vi "Test Micron Driver.vi"() -> ()   [LabVIEW 2024]
uses:
  Micron optics didgitizer configuration.ctl
  Micron Optics Driver/Micron Optics Driver.lvclass
  C:/Git/NHMFL_Core/Libraries/Instruments/VISA Instrument/VISA Instrument.lvclass
  C:/Git/NHMFL_Core/Libraries/Instruments/Instrument Driver/Instrument Driver.lvclass
  Micron sm Digitizer/Micron sm Digitizer.lvclass
  C:/Git/NHMFL_Core/Libraries/Instruments/Micron Optics/Micron Optics Driver/Micron Optics Driver.lvclass
  Micron Hyperion Driver/Micron Hyperion Driver.lvclass
  VISA Instrument/VISA Instrument.lvclass/VISA Instrument.ctl
  Instrument Driver/Instrument Driver.lvclass/Instrument Driver.ctl
  VISA Instrument/Write VISA resource.vi
  Instrument Driver/Write Cycle period.vi
panel:
  out "Waveform Chart":dbl[][](graph)
  in  "Micron Optics Digitizer Configuration":T1={"Post-trigger delay"=0.01, "Post-trigger duration"=0.1, "Rate"=1000000.0, "Reference channel"=-1, "Detection Setting IDs"=[130, 130], "Stream and average"=FALSE, "Address"="10.0.0.55"} {"Rate" format="%#_8pHz"; "Post-trigger duration" format="%#_6ps"; "Post-trigger delay" format="%#_6ps"}
  in  "sm-130  VISA resource":refnum<visa-resource-name>
  in  "Model":enum16{"NONE", "sm-130", "Hyperion"}(ring)=enum."sm-130"
  out "Channel names":string[](array[string])
  in  "stop":bool
  in  "milliseconds to wait":u32=1000
  in  "error in (no error)":errorcluster
  # "Pulse config"
  # "Monitor config"
  # "CH1\n.\n.\n.\n.\n.\nCH4"
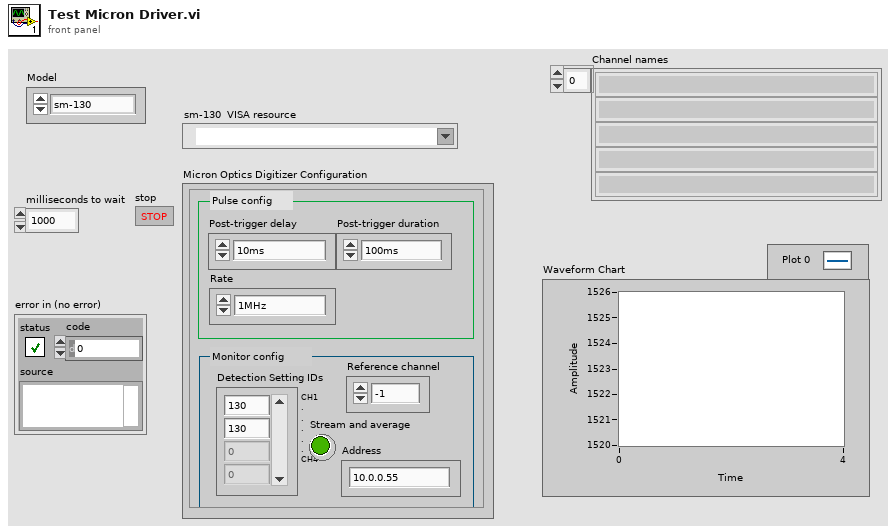
[diagram p1: front panel]
types:
  T1 = typedef "Micron optics didgitizer configuration.ctl" = cluster{"Post-trigger delay":dbl, "Post-trigger duration":dbl, "Rate":dbl, "Reference channel":i32, "Detection Setting IDs":u8[], "Stream and average":bool, "Address":string}
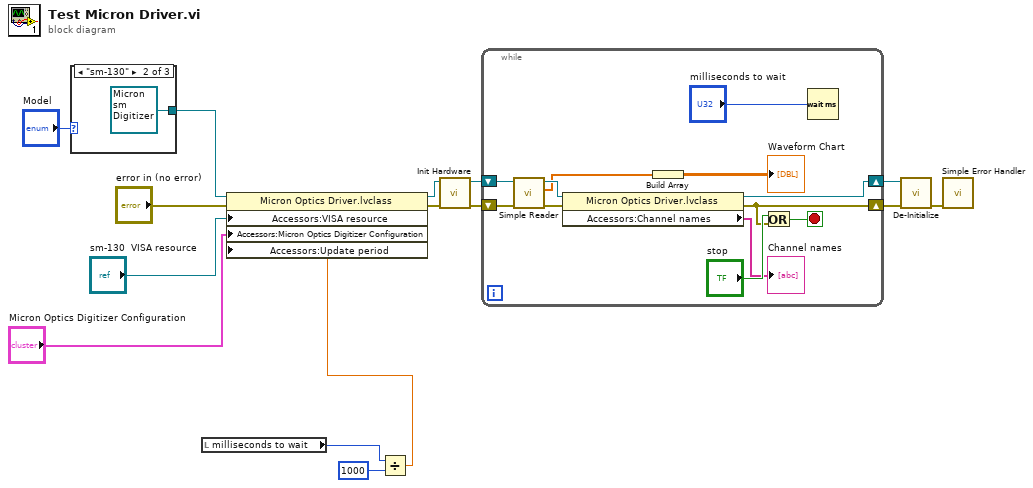
[diagram p0: block diagram]
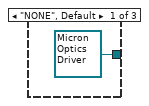
[diagram p2: hidden frame]
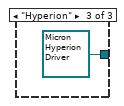
[diagram p3: hidden frame]
diagram:
  n1 = case shown="\"sm-130\"" "Model" {
    tunnel: [refnum<class "Micron Optics Driver.lvclass"> refnum ("Micron Optics Driver.lvclass") refnum<class "Micron sm Digitizer.lvclass"> refnum ("Micron sm Digitizer.lvclass") refnum<class "Micron Hyperion Driver.lvclass"> refnum ("Micron Hyperion Driver.lvclass")] -> w12
    frame "NONE", Default {
    }
    frame "sm-130" {
    }
    frame "Hyperion" {
    }
  }
  n2 = local read "milliseconds to wait"() -> (w3:u32)
  n3 = Divide(x=w3, y=u32 1000) -> (x/y=w1:dbl)
  n4 = property class="Micron Optics Driver.lvclass"(reference=w12, error in="error in (no error)", "Accessors:VISA resource"="sm-130  VISA resource", "Accessors:Micron Optics Digitizer Configuration"="Micron Optics Digitizer Configuration", "Accessors:Update period"=w1) -> (reference out=w9:refnum<class "Micron Optics Driver.lvclass">, error out=w10:errorcluster)
  n5 = call-dynamic "Init Hardware.vi"("error in (no error)"=w10, "Instrument Driver in"=w9) -> ("error out"=w14:errorcluster, "Instrument Driver out"=w15:refnum<class "Micron Optics Driver.lvclass">)  [unwired: 8 in]
  n6 = while {
    shift-right: [w24] -> w6
    shift-left: w15 -> [w27]
    shift-right: [w20] -> w5
    shift-left: w14 -> [w29]
    stop <- w21 stop-if-true
    n7 = call-dynamic "Simple Reader.vi"("error in (no error)"=w29, "Micron Optics Driver in"=w27) -> ("error out"=w28:errorcluster, "Signals"=w22:dbl[], "Micron Optics Driver out"=w25:refnum<class "Micron Optics Driver.lvclass">)  [unwired: 7 in]
    n8 = property class="Micron Optics Driver.lvclass"(reference=w25, error in=w28) -> (reference out=w24:refnum<class "Micron Optics Driver.lvclass">, error out=w20:errorcluster, "Accessors:Channel names"=→"Channel names":string[])
    n9 = Build Array(w22) -> (→"Waveform Chart":dbl[][])
    n10 = Or(x="stop", y=w20) -> (x .or. y?=w21:bool)
    n11 = Wait (ms)(milliseconds to wait="milliseconds to wait") -> ()  [unwired: 1 out]
  }
  n12 = call-dynamic "De-Initialize.vi"("error in (no error)"=w5, "Instrument Driver in"=w6) -> ("error out"=w4:errorcluster)  [unwired: 8 in, 1 out]
  n13 = call <vilib>:"Simple Error Handler.vi"("error in (no error)"=w4) -> ()  [unwired: 4 in, 5 out]
